vi "subRunningSpectrum.vi"(0 "Input Baseband IQ":cdb[](array[numeric]), 1 "averaging parameters":T1={"averaging mode"=enum."No averaging", "weighting mode"=enum."Exponential", "number of averages"=10} {"number of averages" min=1}, 2 "restart averaging":bool, 5 "reset? (F)":bool, 7 "Frame Parameters":T2={"IQ Rate"=0.0, "Frames"=0, "Length of Subset"=0, "Start Index of Subset"=0, "Start Carrier [Hz]"=88500000.0, "Stop Carrier [Hz]"=107700000.0, "Acq Duration [sec]"=0.01} {"Acq Duration [sec]" min=0.0 step=0.001 format="%#.6p"; "Stop Carrier [Hz]" min=50000000.0 max=6000000000.0 step=1000.0 format="%#.15p"; "Start Carrier [Hz]" min=50000000.0 max=6000000000.0 step=1000.0 format="%#.15p"}, 9 "Window Parameters":cluster{"window":T3, "window parameter":dbl}={"window"=2, "window parameter"=nan} {"window" items=["Rectangle"=0, "Hanning"=1, "Hamming"=2, "Blackman-Harris"=3, "Exact Blackman"=4, "Blackman"=5, "Flat Top"=6, "4 Term B-Harris "=7, "7 Term B-Harris"=8, "Low Sidelobe"=9, "Blackman Nuttall"=11, "Triangle"=30, "Bartlett-Hanning"=31, "Bohman"=32, "Parzen"=33, "Welch"=34, "Kaiser"=60, "Dolph-Chebyshev"=61, "Gaussian"=62]}, 11 "error in (no error)":errorcluster, 12 "Iteration":i32) -> (4 "Spectrum to Plot":cluster{"f0":dbl, "df":dbl, "IQ":dbl[]}, 8 "Frame Parameters out":T2={"IQ Rate"=0.0, "Frames"=0, "Length of Subset"=0, "Start Index of Subset"=0, "Start Carrier [Hz]"=88500000.0, "Stop Carrier [Hz]"=107700000.0, "Acq Duration [sec]"=0.01} {"Acq Duration [sec]" min=0.0 step=0.001 format="%#.6p"; "Stop Carrier [Hz]" min=50000000.0 max=6000000000.0 step=1000.0 format="%#.15p"; "Start Carrier [Hz]" min=50000000.0 max=6000000000.0 step=1000.0 format="%#.15p"}, 10 "window properties":cluster{"eq noise BW":dbl, "coherent gain":dbl}, 15 "error out":errorcluster)   [LabVIEW 2015]
uses:
  <vilib>/Analysis/4window.llb/windowTd.ctl
  subFrameParams.ctl
  <vilib>/measure/maspectr.llb/FFT Power Spectrum and PSD for 1 Chan (CDB).vi
  <vilib>/Analysis/4window.llb/Window Properties by Name.vi
  <vilib>/measure/NI_MAPro.lvlib
  <vilib>/Analysis/NI_AALPro.lvlib
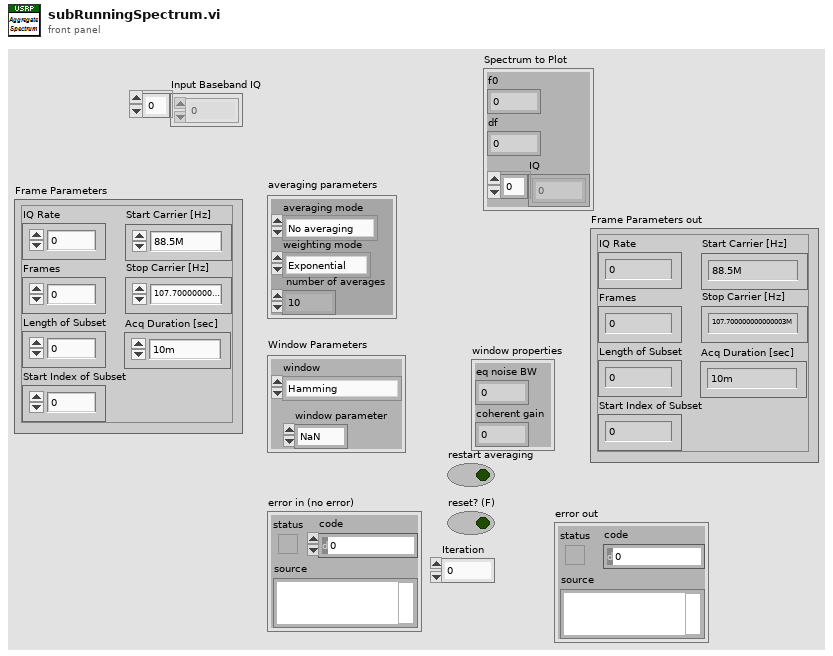
[diagram p1: front panel]
types:
  T1 = cluster{"averaging mode":enum16{"No averaging", "Vector averaging", "RMS averaging", "Peak hold"}, "weighting mode":enum16{"Linear", "Exponential"}, "number of averages":u32}
  T2 = typedef "subFrameParams.ctl" = cluster{"IQ Rate":dbl, "Frames":i32, "Length of Subset":i32, "Start Index of Subset":i32, "Start Carrier [Hz]":dbl, "Stop Carrier [Hz]":dbl, "Acq Duration [sec]":dbl}
  T3 = typedef "NI_AALPro.lvlib/windowTd.ctl" = u32
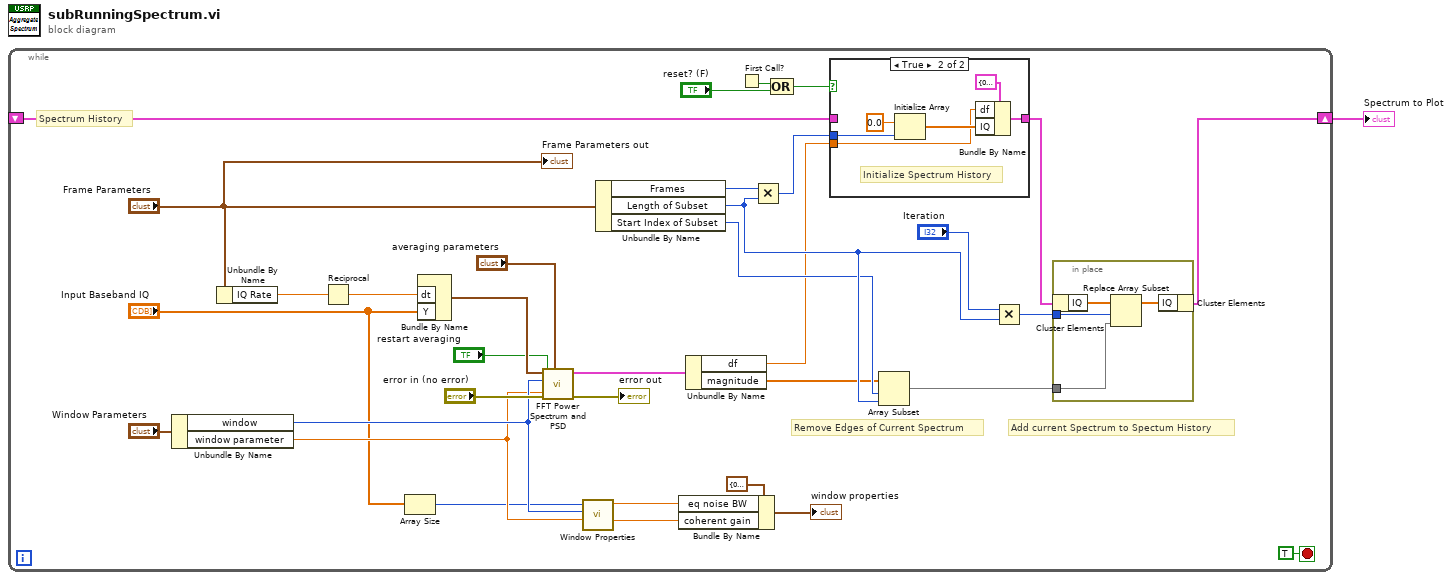
[diagram p0: block diagram]
diagram:
  n1 = while {
    shift-right: [w2] -> w1
    shift-left: _ -> [w34]
    stop <- TRUE stop-if-true
    # "Spectrum History"
    # "Remove Edges of Current Spectrum"
    # "Add current Spectrum to Spectum History"
    n2 = Unbundle By Name("Window Parameters") -> ("window"=w12:T3, "window parameter"=w11:dbl)
    n3 = Unbundle By Name("Frame Parameters") -> ("IQ Rate"=w3:dbl)
    n4 = Reciprocal(x=w3) -> (1/x=w21:dbl)
    n5 = Array Size(array="Input Baseband IQ") -> (size(s)=w5:i32)
    n6 = Bundle By Name("dt"=w21, "Y"="Input Baseband IQ") -> (w20:waveform(cdb))  [unwired: 1 in]
    n7 = call-poly <vilib>:"FFT Power Spectrum and PSD.vi"("window parameter"=w11, "averaging parameters"="averaging parameters", "restart averaging (F)"="restart averaging", "error in (no error)"="error in (no error)", "window"=w12, "time signal"=w20) -> ("error out"=→"error out":errorcluster, "Power Spectrum / PSD"=w17:cluster{"f0":dbl, "df":dbl, "magnitude":dbl[]})  [unwired: 2 in, 2 out]
    n8 = call-poly <vilib>:"Window Properties.vi"("window parameter"=w11, "window"=w12, "size"=w5) -> ("coherent gain"=w7:dbl, "eq noise BW"=w8:dbl)  [unwired: 6 in, 1 out]
    n9 = Unbundle By Name("Frame Parameters") -> ("Frames"=w32:i32, "Length of Subset"=w31:i32, "Start Index of Subset"=w29:i32)
    n10 = Bundle By Name(cluster=cluster{"eq noise BW":dbl, "coherent gain":dbl} {"eq noise BW"=0.0, "coherent gain"=0.0} ("window properties"), "eq noise BW"=w8, "coherent gain"=w7) -> (→"window properties":cluster{"eq noise BW":dbl, "coherent gain":dbl})
    n11 = Unbundle By Name(w17) -> ("df"=w16:dbl, "magnitude"=w15:dbl[])
    n12 = First Call?() -> (First Call?: T/F=w22:bool)
    n13 = Multiply(x=w32, y=w31) -> (x*y=w35:i32)
    n14 = Compound Arithmetic op=OR(w22, "reset? (F)") -> (w24:bool)
    n15 = case shown="True" w24 {
      tunnel: w35 -> [_ w45]
      tunnel: [w40 w42] -> w28
      tunnel: w34 -> [w40 _]
      tunnel: w16 -> [_ w43]
      frame False {
      }
      frame True {
        # "Initialize Spectrum History"
        n16 = Initialize Array(0.0 ("Numeric"), w45) -> (w44:dbl[])
        n17 = Bundle By Name(cluster=cluster{"f0":dbl, "df":dbl, "IQ":dbl[]} {"f0"=0.0, "df"=0.0, "IQ"=[]} ("Spectrum to Plot"), "df"=w43, "IQ"=w44) -> (w42:cluster{"f0":dbl, "df":dbl, "IQ":dbl[]})
      }
    }
    n18 = Array Subset(array=w15, index=w29, length=w31) -> (w26:dbl[])
    n19 = Multiply(x="Iteration", y=w31) -> (x*y=w27:i32)
    n20 = in-place {
      in-place-border: w27 -> [w39]
      in-place-border: w26 -> [w38]
      n21 = in-place-cluster #1(w28) -> ("IQ"=w37:dbl[])
      n22 = Replace Array Subset(array=w37, new element=w38, index=w39) -> (w36:dbl[])
      n23 = in-place-cluster #1("IQ"=w36) -> (w2:cluster{"f0":dbl, "df":dbl, "IQ":dbl[]})
    }
    "Frame Parameters out" <- "Frame Parameters"
  }
  "Spectrum to Plot" <- w1
